vi "GFITS_GetDataTypes.vi"(9 "type":string, 10 "keys":string[][](array[string])) -> (1 "keys out":string[][](array[string]), 2 "datatypes":i32[](array[numeric]))   [LabVIEW 2016]
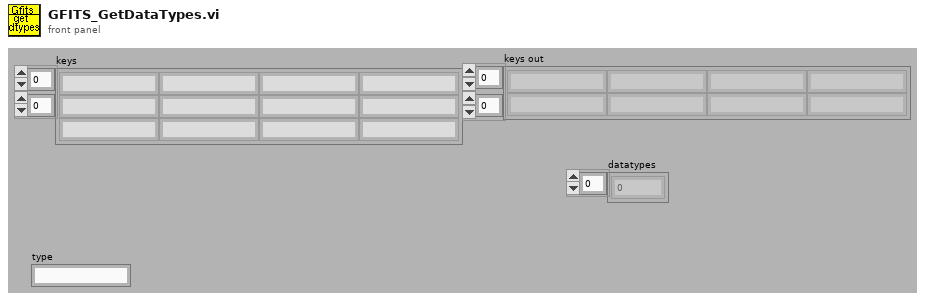
[diagram p1: front panel]
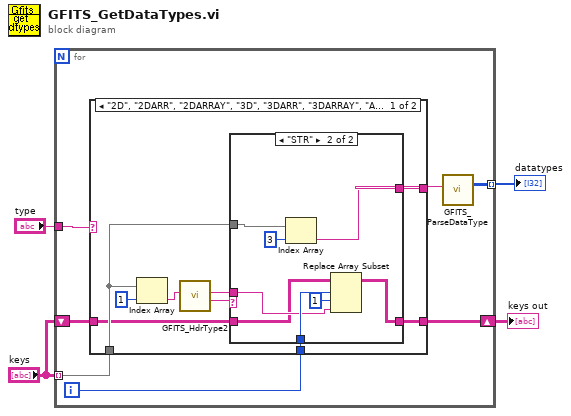
[diagram p0: block diagram]
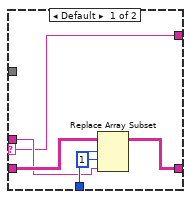
[diagram p2: hidden frame]
diagram:
  n1 = for {
    tunnel: "type" -> [w11]
    tunnel: "keys" -> [w8] mode=indexing
    tunnel: [w9] -> w3 mode=indexing
    shift-right: [w6] -> w1
    shift-left: "keys" -> [w7]
    i -> [w5]
    n2 = case shown="\"2D\", \"2DARR\", \"2DARRAY\", \"3D\", \"3DARR\", \"3DARRAY\", \"ARR\"" w11 {
      selector: w11 -> [_ w36]
      tunnel: [w12 w36] -> w10
      tunnel: w8 -> [w19 _]
      tunnel: w7 -> [w15 w35]
      tunnel: [w14 w35] -> w6
      tunnel: w5 -> [w13 _]
      frame "2D", "2DARR", "2DARRAY", "3D", "3DARR", "3DARRAY", "ARR" {
        n3 = Index Array(array=w19, index=1) -> (element=w18:string)
        n4 = call "GFITS_HdrType2.vi"("keyval"=w18) -> ("type"=w17:string, "keyval out"=w16:string)  [unwired: 9 out]
        n5 = case shown="\"STR\"" w17 {
          selector: w17 -> [w21 _]
          tunnel: w19 -> [_ w33]
          tunnel: w16 -> [w22 w29]
          tunnel: w15 -> [w26 w28]
          tunnel: [w25 w27] -> w14
          tunnel: w13 -> [w24 w31]
          tunnel: [w21 w32] -> w12
          frame Default {
            n6 = Replace Array Subset(array=w26, new element=w22, index (row)=w24, index (col)=1 ("disabled index (col)")) -> (w25:string[][])
          }
          frame "STR" {
            n7 = Index Array(array=w33, index=3) -> (element=w32:string)
            n8 = Replace Array Subset(array=w28, new element=w29, index (row)=w31, index (col)=1 ("disabled index (col)")) -> (w27:string[][])
          }
        }
      }
      frame Default {
      }
    }
    n9 = call "GFITS_ParseDataType.vi"("string type"=w10) -> ("numeric type"=w9:i32)  [unwired: 10 out]
  }
  "datatypes" <- w3
  "keys out" <- w1
